vi "incrementBroadcastCounter.vi"(8 "error in (no error)":errorcluster, 11 "Subnet in":refnum<class "ISubnet.lvclass">) -> (0 "error out":errorcluster, 3 "Subnet out":refnum<class "ISubnet.lvclass">)   [LabVIEW 2015, in "ISubnet.lvclass"]
uses:
  ISubnet.lvclass
  ISubnet.lvclass/ISubnet.ctl
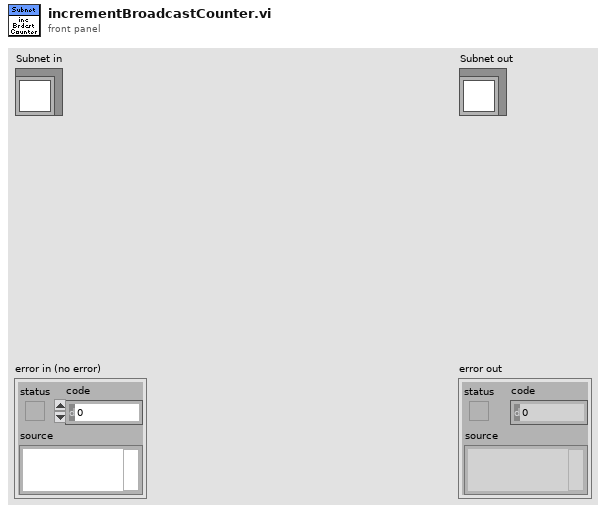
[diagram p1: front panel]
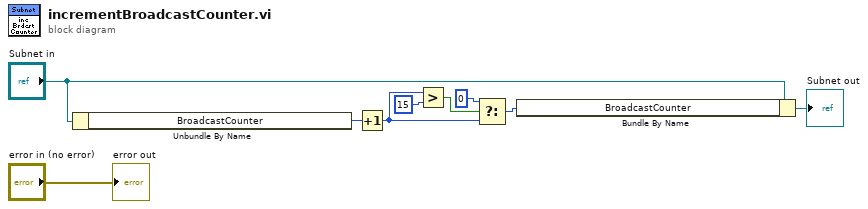
[diagram p0: block diagram]
diagram:
  n1 = Unbundle By Name("Subnet in") -> ("BroadcastCounter"=w9:u8)
  n2 = Increment(x=w9) -> (x+1=w6:u8)
  n3 = Greater?(x=w6, y=u16 15) -> (0:w7:bool)
  n4 = Select(t=u16 0, s=w7, f=w6) -> (s? t:f=w3:u16)
  n5 = Bundle By Name(cluster="Subnet in", "BroadcastCounter"=w3) -> (→"Subnet out":refnum<class "ISubnet.lvclass">)
  "error out" <- "error in (no error)"
